vi "filterBigJumps.vi"(4 "FPS":dbl, 6 "threshold value":dbl, 10 "prev final value":dbl, 11 "calc value":dbl) -> (3 "filtered value":dbl)   [LabVIEW 2020]
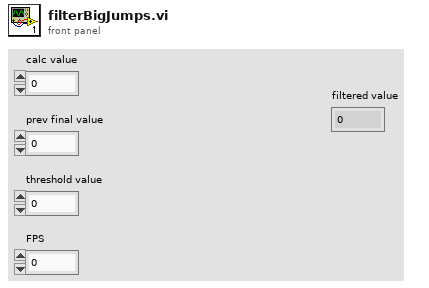
[diagram p1: front panel]
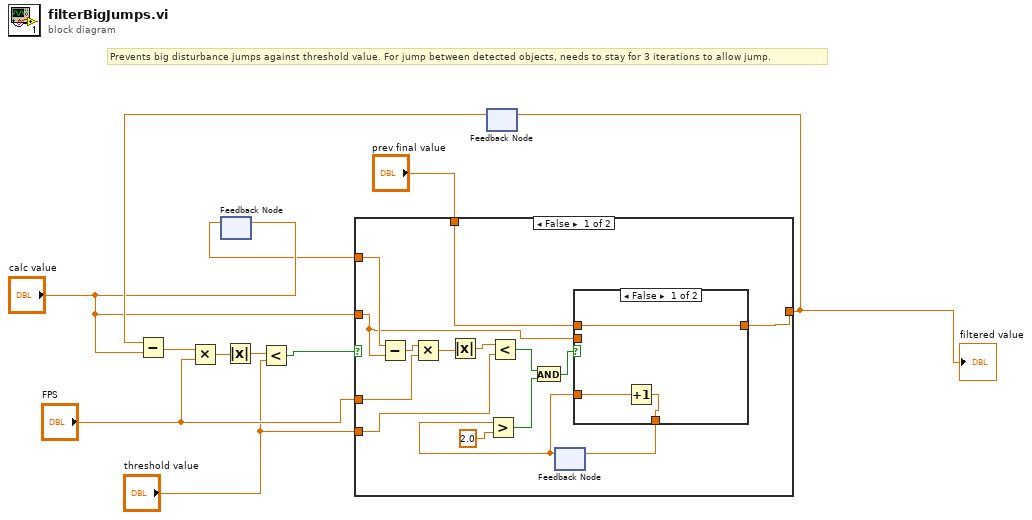
[diagram p0: block diagram]
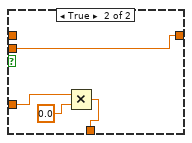
[diagram p2: hidden frame]
diagram:
  # "Prevents big disturbance jumps against threshold value. For jump between detected objects, needs to stay for 3 iterations to allow jump."
  n1 = feedback #1() -> (w3:dbl)  [unwired: 1 in]
  n2 = feedback-in #1("calc value") -> ()
  n3 = feedback #2() -> (w8:dbl)  [unwired: 1 in]
  n4 = Subtract(x=w8, y="calc value") -> (x-y=w11:dbl)
  n5 = Multiply(x=w11, y="FPS") -> (x*y=w10:dbl)
  n6 = Absolute Value(x=w10) -> (abs(x)=w9:dbl)
  n7 = Less?(x=w9, y="threshold value") -> (x < y?=w7:bool)
  n8 = case shown="False" w7 {
    tunnel: [w18 w34] -> w1
    tunnel: "calc value" -> [w16 w34]
    tunnel: w3 -> [w19 _]
    tunnel: "prev final value" -> [w17 _]
    tunnel: "FPS" -> [w14 _]
    tunnel: "threshold value" -> [w12 _]
    frame False {
      n9 = Subtract(x=w19, y=w16) -> (x-y=w26:dbl)
      n10 = Multiply(x=w26, y=w14) -> (x*y=w25:dbl)
      n11 = Absolute Value(x=w25) -> (abs(x)=w24:dbl)
      n12 = Less?(x=w24, y=w12) -> (x < y?=w23:bool)
      n13 = feedback #3() -> (w13:dbl)  [unwired: 1 in]
      n14 = Greater?(x=w13, y=2.0) -> (0:w22:bool)
      n15 = And(x=w23, y=w22) -> (x .and. y?=w20:bool)
      n16 = case shown="False" w20 {
        tunnel: [w29 w33] -> w18
        tunnel: w17 -> [w29 _]
        tunnel: w16 -> [_ w33]
        tunnel: [w28 w30] -> w15
        tunnel: w13 -> [w27 w31]
        frame False {
          n17 = Increment(x=w27) -> (x+1=w28:dbl)
        }
        frame True {
          n18 = Multiply(x=w31, y=0.0) -> (x*y=w30:dbl)
        }
      }
      n19 = feedback-in #3(w15) -> ()
    }
    frame True {
    }
  }
  "filtered value" <- w1
  n20 = feedback-in #2(w1) -> ()
